vi "Powerup Test.vi"(11 "PowerFail":bool) -> (0 "error out":errorcluster, 3 "Result":bool)   [LabVIEW 2011]
doc: "Apply power to the motherboard and verify that it powers on successfully."
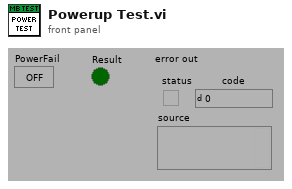
[diagram p1: front panel]
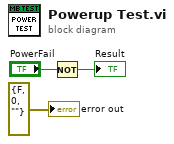
[diagram p0: block diagram]
diagram:
  n1 = Not(x="PowerFail") -> (.not. x?=→"Result":bool)
  "error out" <- errorcluster {"status"=FALSE, "code"=0, "source"=""} ("error out")
